vi "GetElements(Multiple).vi"(7 "Qualified Name":string, 8 "error in (no error)":errorcluster, 10 "keys":string[](array[string]), 11 "ConfigManager.Text.INI in":refnum<class "ConfigManager.Text.INI.lvclass">) -> (0 "error out":errorcluster, 1 "Values":string[](array[string]), 2 "Keys":string[](array[string]), 3 "ConfigManager.Text.INI out":refnum<class "ConfigManager.Text.INI.lvclass">, 4 "Found":bool[](array[boolean]))   [LabVIEW 2013, in "CfgManager.Text.lvlib" / "ConfigManager.Text.INI.lvclass"]
uses:
  ConfigManager.Text.INI.lvclass
  Manager.Text/ConfigManager.Text.lvclass
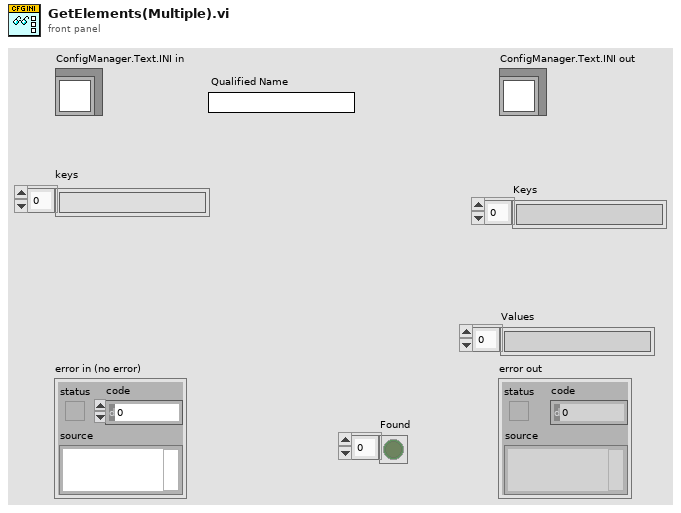
[diagram p1: front panel]
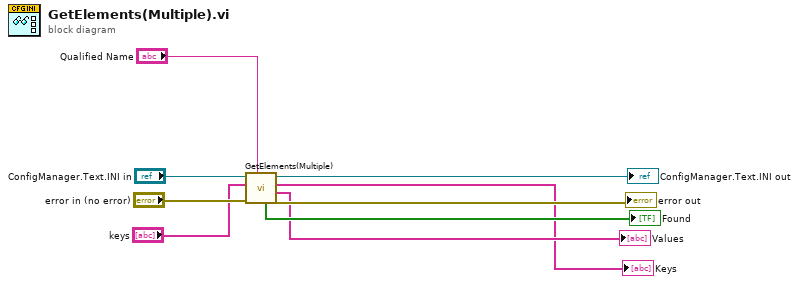
[diagram p0: block diagram]
diagram:
  n1 = call-parent "GetElements(Multiple).vi"("Qualified Name"="Qualified Name", "error in (no error)"="error in (no error)", "keys"="keys", "ConfigManager.Text in"="ConfigManager.Text.INI in") -> ("error out"=→"error out":errorcluster, "Values"=→"Values":string[], "Keys"=→"Keys":string[], "ConfigManager.Text out"=→"ConfigManager.Text.INI out":refnum<class "ConfigManager.Text.INI.lvclass">, "Found"=→"Found":bool[])  [unwired: 3 in]
